vi "getData.vi"(8 "error in (no error)":errorcluster, 11 "ScriptEvent in":refnum<class "ScriptEvent.lvclass">) -> (0 "error out":errorcluster, 1 "dataType":T1(ring), 2 "data":T2, 3 "ScriptEvent out":refnum<class "ScriptEvent.lvclass">)   [LabVIEW 2009, in "Tools.lvlib" / "Scripting.lvlib" / "ScriptEvent.lvclass"]
uses:
  ScriptEvent.lvclass
  DatabaseHelpers/Database Objects/Channel/Channel.lvclass
  ScriptEvent.lvclass/ScriptEvent.ctl
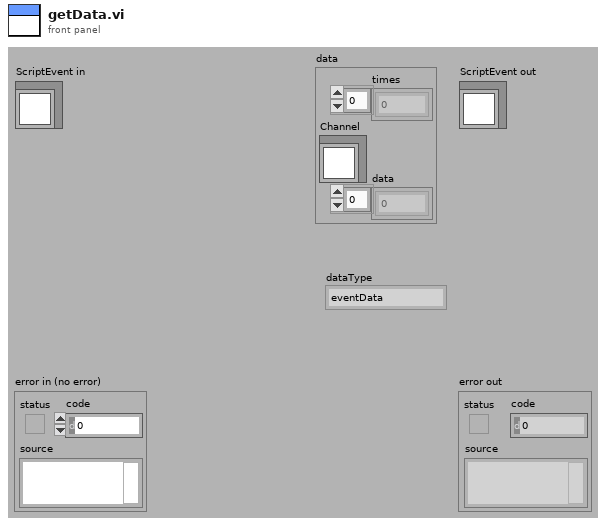
[diagram p1: front panel]
types:
  T1 = enum16{"eventData", "singleToneData", "fileData"}
  T2 = cluster{"times":dbl[], "Channel":refnum<class "Channel.lvclass">, "data":dbl[]}
  T3 = cluster{dbl[], "Channel":refnum<class "Channel.lvclass">, dbl[]}
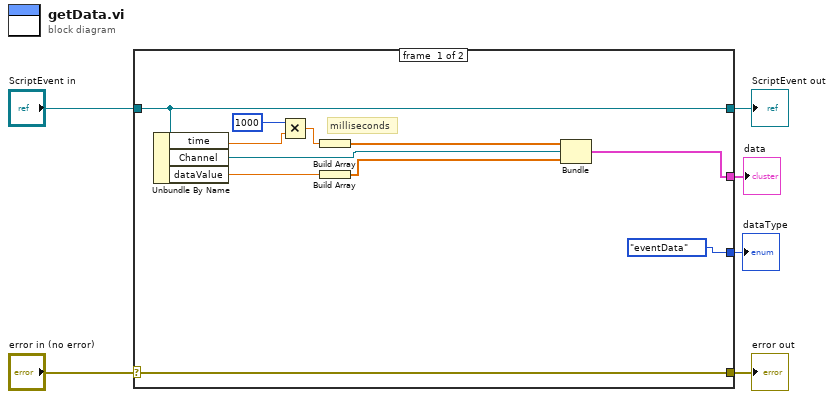
[diagram p0: block diagram]
diagram:
  n1 = case shown="No Error" "error in (no error)" {
    selector: "error in (no error)" -> [w11 w19]
    tunnel: [w11 w19] -> w5
    tunnel: [w17 w18] -> w3
    tunnel: "ScriptEvent in" -> [w17 w18]
    tunnel: [w14 _] -> w2
    tunnel: [T1."eventData" ("dataType") _] -> w1
    frame #0 {
      # "milliseconds"
      n2 = Unbundle By Name(w17) -> ("time"=w10:dbl, "Channel"=w12:refnum<class "Channel.lvclass">, "dataValue"=w16:dbl)
      n3 = Multiply(x=1000, y=w10) -> (x*y=w9:dbl)
      n4 = Build Array(w9) -> (w13:dbl[])
      n5 = Build Array(w16) -> (w15:dbl[])
      n6 = Bundle(w13, "Channel"=w12, w15) -> (w14:T3)  [unwired: 1 in]
    }
    frame #1 {
    }
  }
  "error out" <- w5
  "ScriptEvent out" <- w3
  "data" <- w2
  "dataType" <- w1
